vi "Select Channels GUI.vi"(8 "error in (no error)":errorcluster, 11 "SimpleGraphEditorPanel in":refnum<class "SimpleGraphEditorPanel.lvclass">) -> (0 "error out":errorcluster, 2 "Cancelled":bool, 3 "SimpleGraphEditorPanel out":refnum<class "SimpleGraphEditorPanel.lvclass">)   [LabVIEW 2020, in "VolatusGUIControls.lvlib" / "SimpleGraphEditorPanel.lvclass"]
uses:
  SimpleGraphEditorPanel.lvclass
  C:/dev/lv20CE/relink/volatus-gui-controls/VolatusGUIEditorCore/ElementEditorPanel/ElementEditorPanel.lvclass
  JSON Props.ctl
  SimpleGraphEditorPanel.lvclass/SimpleGraphEditorPanel.ctl
  lv-autocomplete/AutoComplete/AutoComplete/AutoComplete.lvclass/AutoComplete.ctl
  23eae216-a268-49b7-aef0-9a1c86c85678.vi
  <vilib>/JDP Science/JSONtext/JSON text to Variant.vi
  lv-autocomplete/AutoComplete/Launch Autocomplete Handler.vi
  <vilib>/JDP Science/JSONtext/LVClass Serializer/JSONtext LVClass Serializer.lvclass
  lv-autocomplete/AutoComplete/AutoComplete/AutoComplete.lvclass
  VolatusGUIEditorCore/ElementEditorPanel/ElementEditorPanel.lvclass
  VolatusGUIControls.lvlib
  VolatusGUIEditorCore/VolatusGUIEditorCore.lvlib
panel:
  in  "Listbox":i32(listbox)
  in  "Down":bool
  in  "Up":bool
  in  "Cancel":bool
  in  "OK":bool
  in  "Configured Channels":i32(listbox)
  in  "Add":bool
  in  "Channel to Add":string
  # "Double-click to remove"
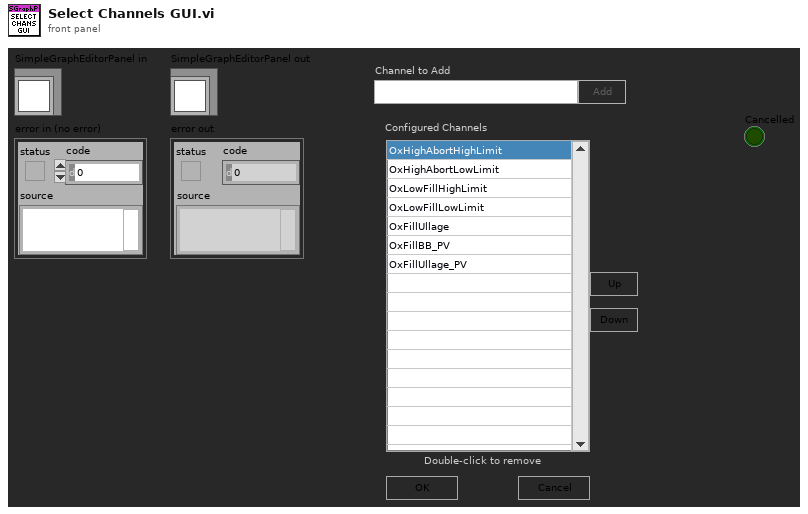
[diagram p1: front panel]
types:
  T1 = enum8{"Enabled", "Disabled", "Disabled and Grayed Out"}
  T2 = typedef "VolatusGUIControls.lvlib/SimpleGraphEditorPanel.lvclass/JSON Props.ctl" = cluster{"Channels":string[], "Buffer_Length":i32, "Redraw_Period_s":dbl, "Duration_s":i32}
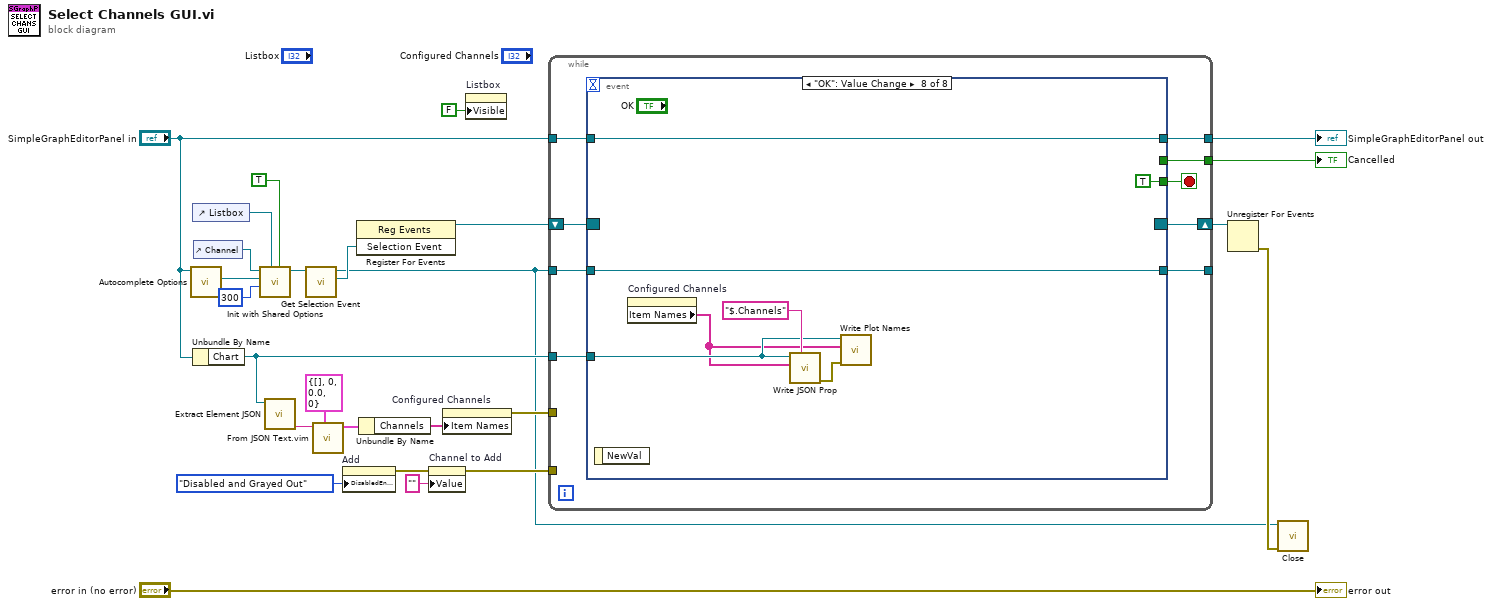
[diagram p0: block diagram]
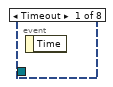
[diagram p2: hidden frame]
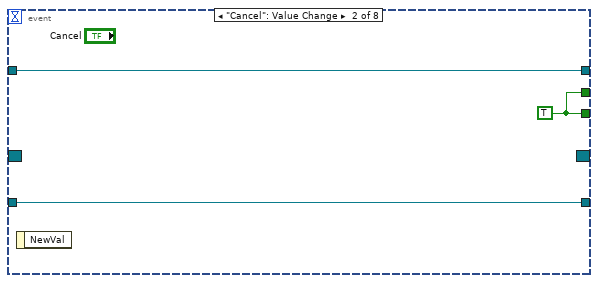
[diagram p3: hidden frame]
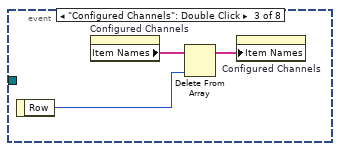
[diagram p4: hidden frame]
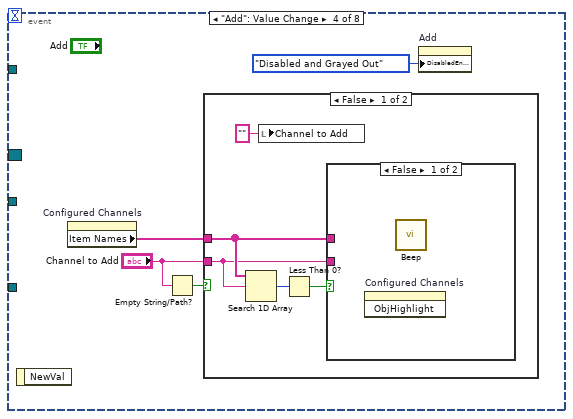
[diagram p5: hidden frame]
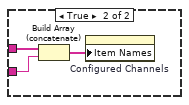
[diagram p6: hidden frame]
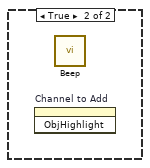
[diagram p7: hidden frame]
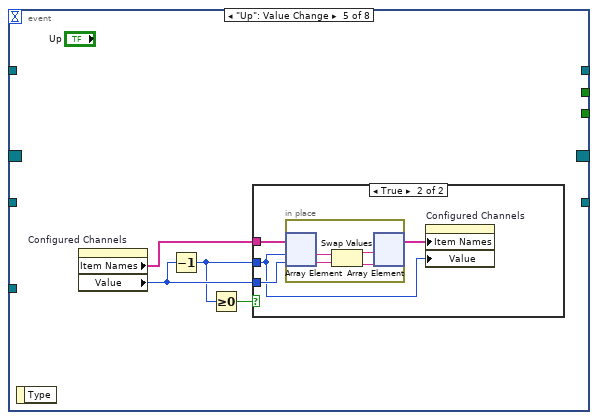
[diagram p8: hidden frame]
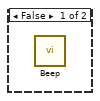
[diagram p9: hidden frame]
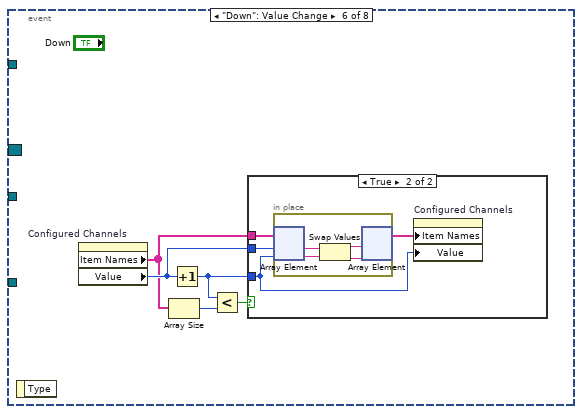
[diagram p10: hidden frame]
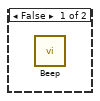
[diagram p11: hidden frame]
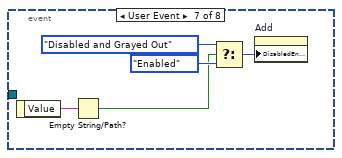
[diagram p12: hidden frame]
diagram:
  n1 = call "Autocomplete Options.vi"("ElementEditorPanel in"="SimpleGraphEditorPanel in") -> ("Autocomplete Options"=w25:refnum<class "Shared Options.lvclass">)  [unwired: 10 in]
  n2 = control-ref of="Listbox"() -> (w5:refnum<vi>)
  n3 = Unbundle By Name("SimpleGraphEditorPanel in") -> ("Chart"=w6:refnum<vi>)
  n4 = control-ref of="Channel"() -> (w24:refnum<vi>)
  n5 = call "Init with Shared Options.vi"("Autohide ListBox (F)"=TRUE, "ListBox Refnum (Popup)"=w5, "Height (200)"=i16 300, "Shared Options"=w25, "Str Refnum"=w24) -> ("AutoComplete out"=w22:refnum<class "AutoComplete.lvclass">)  [unwired: 5 in, 1 out]
  n6 = call "Extract Element JSON.vi"("Ctl Refnum in"=w6) -> ("JSON"=w15:string)  [unwired: 7 in, 3 out]
  n7 = call "Get Selection Event.vi"("AutoComplete in"=w22) -> ("Selection Event"=w21:refnum<user-event>, "AutoComplete"=w1:refnum<class "AutoComplete.lvclass">)  [unwired: 9 in]
  n8 = call "From JSON Text.vim"("Data Type and Default Value"=T2 {"Channels"=[], "Buffer_Length"=0, "Redraw_Period_s"=0.0, "Duration_s"=0} ("JSON Props"), "JSON"=w15) -> ("Data out"=w13:T2)  [unwired: 8 in, 1 out]
  n9 = property on="Add" class="Bool"("DisabledEnum"=T1."Disabled and Grayed Out" ("Disabled")) -> (error out=w8:errorcluster)  [unwired: 2 in, 1 out]
  n10 = register-events(w21) -> (reference out=w20:refnum<event-registration>)  [unwired: 2 in, 1 out]
  n11 = Unbundle By Name(w13) -> ("Channels"=w12:string[])
  n12 = property on="Channel to Add" class="Str"(error in=w8, "Value"="" ("Channel to Add")) -> (error out=w7:errorcluster)  [unwired: 1 in, 1 out]
  n13 = property on="Configured Channels" class="LstBox (strict)"("Item Names"=w12) -> (error out=w10:errorcluster)  [unwired: 2 in, 1 out]
  n14 = property on="Listbox" class="LstBox (strict)"("Visible"=FALSE) -> ()  [unwired: 2 in, 2 out]
  n15 = while {
    tunnel: "SimpleGraphEditorPanel in" -> [w34]
    shift-right: [w32] -> w19
    shift-left: w20 -> [w35]
    tunnel: w1 -> [w33]
    tunnel: [w31] -> w18
    tunnel: [w29] -> _
    tunnel: [w28] -> w17
    tunnel: w10 -> [_]
    tunnel: w7 -> [_]
    tunnel: w6 -> [w27]
    stop <- w30 stop-if-true
    n16 = event shown="[7] \"OK\": Value Change" {
      selector: w35 -> [_ _ _ _ _ _ _ _]
      dyn-events: [_ _ _ _ _ _ _ _] -> w32
      timeout: _ -> [_ _ _ _ _ _ _ _]
      tunnel: w34 -> [_ w38 _ _ _ _ _ w90]
      tunnel: w33 -> [_ w37 _ _ _ _ _ w89]
      tunnel: [_ w38 _ _ _ _ _ w90] -> w31
      tunnel: [_ w36 _ _ _ _ _ TRUE] -> w30
      tunnel: [_ w37 _ _ _ _ _ w89] -> w29
      tunnel: [_ w36 _ _ _ _ _ _] -> w28
      tunnel: w27 -> [_ _ _ _ _ _ _ w86]
      event Timeout {
        n17 = event-data() -> ()  [unwired: 1 in, 1 out]
      }
      event "Cancel": Value Change {
        w36 = TRUE
        n18 = event-data() -> ()  [unwired: 1 in, 1 out]
      }
      event "Configured Channels": Double Click {
        n19 = event-data() -> ("Row"=w40:i32)  [unwired: 1 in]
        n20 = property on="Configured Channels" class="LstBox (strict)"() -> ("Item Names"=w41:string[])  [unwired: 2 in, 2 out]
        n21 = Delete From Array(array=w41, index=w40) -> (array with subset deleted=w39:string[])  [unwired: 1 in, 1 out]
        n22 = property on="Configured Channels" class="LstBox (strict)"("Item Names"=w39) -> ()  [unwired: 2 in, 2 out]
      }
      event "Add": Value Change {
        n23 = event-data() -> ()  [unwired: 1 in, 1 out]
        n24 = property on="Configured Channels" class="LstBox (strict)"() -> ("Item Names"=w42:string[])  [unwired: 2 in, 2 out]
        n25 = Empty String/Path?(string/path="Channel to Add") -> (empty?=w44:bool)
        n26 = case shown="False" w44 {
          tunnel: "Channel to Add" -> [w49 _]
          tunnel: w42 -> [w50 _]
          frame False {
            n27 = Search 1D Array(1D array=w50, element=w49) -> (index of element=w48:i32)  [unwired: 1 in]
            n28 = local write "Channel to Add"("" ("Channel to Add")) -> ()
            n29 = Less Than 0?(x=w48) -> (x < 0?=w47:bool)
            n30 = case shown="False" w47 {
              tunnel: w50 -> [_ w52]
              tunnel: w49 -> [_ w51]
              frame False {
                n31 = invoke on="Configured Channels" class="LstBox (strict)" method="ObjHighlight"() -> ()  [unwired: 3 in, 3 out]
                n32 = call <vilib>:"Beep.vi"() -> ()  [unwired: 12 in]
              }
              frame True {
                n33 = Build Array (concatenate)(w52, w51) -> (w53:string[])
                n34 = property on="Configured Channels" class="LstBox (strict)"("Item Names"=w53) -> ()  [unwired: 2 in, 2 out]
              }
            }
          }
          frame True {
            n35 = invoke on="Channel to Add" class="Str" method="ObjHighlight"() -> ()  [unwired: 3 in, 3 out]
            n36 = call <vilib>:"Beep.vi"() -> ()  [unwired: 12 in]
          }
        }
        n37 = property on="Add" class="Bool"("DisabledEnum"=T1."Disabled and Grayed Out" ("Disabled")) -> ()  [unwired: 2 in, 2 out]
      }
      event "Up": Value Change {
        n38 = event-data() -> ()  [unwired: 1 in, 1 out]
        n39 = property on="Configured Channels" class="LstBox (strict)"() -> ("Item Names"=w57:string[], "Value"=w56:i32)  [unwired: 2 in, 2 out]
        n40 = Decrement(x=w56) -> (x-1=w55:i32)
        n41 = Greater Or Equal To 0?(x=w55) -> (x >= 0?=w54:bool)
        n42 = case shown="True" w54 {
          tunnel: w57 -> [_ w61]
          tunnel: w56 -> [_ w60]
          tunnel: w55 -> [_ w58]
          frame False {
            n43 = call <vilib>:"Beep.vi"() -> ()  [unwired: 12 in]
          }
          frame True {
            n44 = in-place {
              n45 = in-place-array #1(w61, w58, w60) -> (w65:string, w64:string)
              n46 = Swap Values(12:w65, 14:w64) -> (1:w63:string, 3:w62:string)  [unwired: 1 in]
              n47 = in-place-array #1(w63, w62) -> (w59:string[])  [unwired: 2 out]
            }
            n48 = property on="Configured Channels" class="LstBox (strict)"("Item Names"=w59, "Value"=w58) -> ()  [unwired: 2 in, 2 out]
          }
        }
      }
      event "Down": Value Change {
        n49 = event-data() -> ()  [unwired: 1 in, 1 out]
        n50 = property on="Configured Channels" class="LstBox (strict)"() -> ("Item Names"=w69:string[], "Value"=w70:i32)  [unwired: 2 in, 2 out]
        n51 = Array Size(array=w69) -> (size(s)=w68:i32)
        n52 = Increment(x=w70) -> (x+1=w67:i32)
        n53 = Less?(x=w67, y=w68) -> (x < y?=w66:bool)
        n54 = case shown="True" w66 {
          tunnel: w70 -> [_ w73]
          tunnel: w69 -> [_ w72]
          tunnel: w67 -> [_ w71]
          frame False {
            n55 = call <vilib>:"Beep.vi"() -> ()  [unwired: 12 in]
          }
          frame True {
            n56 = in-place {
              n57 = in-place-array #2(w72, w73, w71) -> (w78:string, w77:string)
              n58 = Swap Values(12:w78, 14:w77) -> (1:w76:string, 3:w75:string)  [unwired: 1 in]
              n59 = in-place-array #2(w76, w75) -> (w74:string[])  [unwired: 2 out]
            }
            n60 = property on="Configured Channels" class="LstBox (strict)"("Item Names"=w74, "Value"=w71) -> ()  [unwired: 2 in, 2 out]
          }
        }
      }
      event User Event {
        n61 = event-data() -> ("Value"=w83:string)  [unwired: 1 in]
        n62 = Empty String/Path?(string/path=w83) -> (empty?=w80:bool)
        n63 = Select(t=T1."Disabled and Grayed Out" ("Disabled"), s=w80, f=T1."Enabled") -> (s? t:f=w79:T1)
        n64 = property on="Add" class="Bool"("DisabledEnum"=w79) -> ()  [unwired: 2 in, 2 out]
      }
      event "OK": Value Change {
        n65 = event-data() -> ()  [unwired: 1 in, 1 out]
        n66 = property on="Configured Channels" class="LstBox (strict)"() -> ("Item Names"=w84:string[])  [unwired: 2 in, 2 out]
        n67 = call "Write JSON Prop.vi"("JSON Path"="$.Channels", "Value"=w84, "Ctl Refnum in"=w86) -> ("error out"=w85:errorcluster)  [unwired: 7 in, 1 out]
        n68 = call "Write Plot Names.vi"("error in (no error)"=w85, "Names"=w84, "Graph in"=w86) -> ()  [unwired: 7 in, 2 out]
      }
    }
  }
  "SimpleGraphEditorPanel out" <- w18
  "Cancelled" <- w17
  n69 = Unregister For Events(event registration refnum=w19) -> (error out=w2:errorcluster)  [unwired: 1 in]
  n70 = call "Close.vi"("error in (no error)"=w2, "AutoComplete in"=w1) -> ()  [unwired: 9 in, 1 out]
  "error out" <- "error in (no error)"
